vi "Configure AC Frequency Limit.vi"(8 "error in":errorcluster, 9 "Level(HZ)":dbl=1.0 min=0.01 format="%.2g", 10 "Type":u16(ring) items=["Max", "Min"], 11 "VISA resource name":refnum<visa-resource-name>) -> (0 "error out":errorcluster, 3 "VISA resource name out":refnum<visa-resource-name>)   [LabVIEW 2020, in "IT-M7700.lvlib"]
doc: "This command is used to set the minimum/maximum FREQ of AC.\n<b>Type</b>\n0: MAX\n1: MIN\n<b>Level(HZ)</b>\nMIN-MAX"
uses:
  <instrlib>/IT-M7700/IT-M7700.lvlib
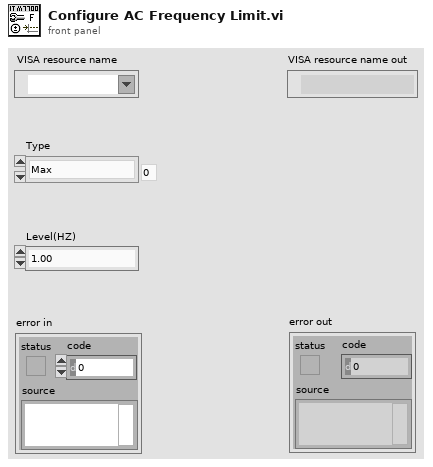
[diagram p1: front panel]
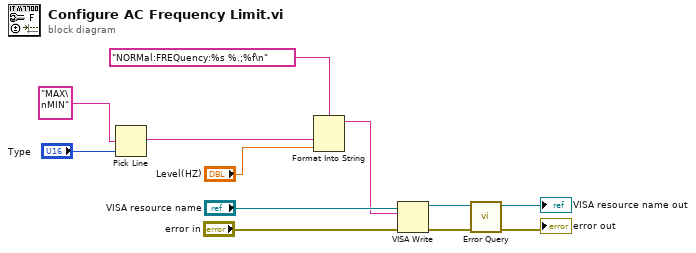
[diagram p0: block diagram]
diagram:
  n1 = Pick Line(multi-line string="MAX\nMIN", line index="Type") -> (output string=w1:string)  [unwired: 1 in]
  n2 = Format Into String(format string="NORMal:FREQuency:%s %.;%f\n", w1, "Level(HZ)") -> (resulting string=w10:string)  [unwired: 2 in, 1 out]
  n3 = VISA Write(VISA resource name="VISA resource name", write buffer=w10, error in (no error)="error in") -> (VISA resource name out=w9:refnum<visa-resource-name>, error out=w8:errorcluster)  [unwired: 1 out]
  n4 = call <instrlib>:"Error Query.vi"("error in"=w8, "VISA resource name"=w9) -> ("error out"=→"error out":errorcluster, "VISA resource name out"=→"VISA resource name out":refnum<visa-resource-name>)  [unwired: 6 in, 2 out]
